vi "Number list to array.vi"(10 "Full names prefix":string, 11 "Number list":string) -> (2 "Full names":string[](array[string]), 3 "Number list array":i32[](array[numeric]))   [LabVIEW 2019]
panel:
  out "substring":string
  out "number":i32
  out "offset past number":i32
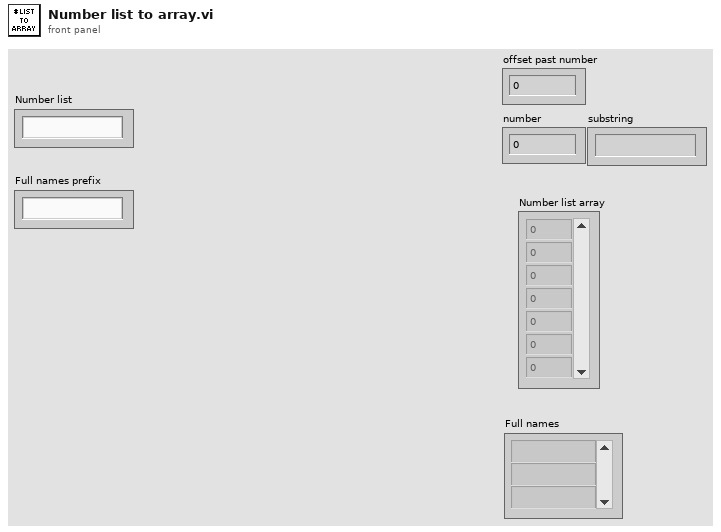
[diagram p1: front panel]
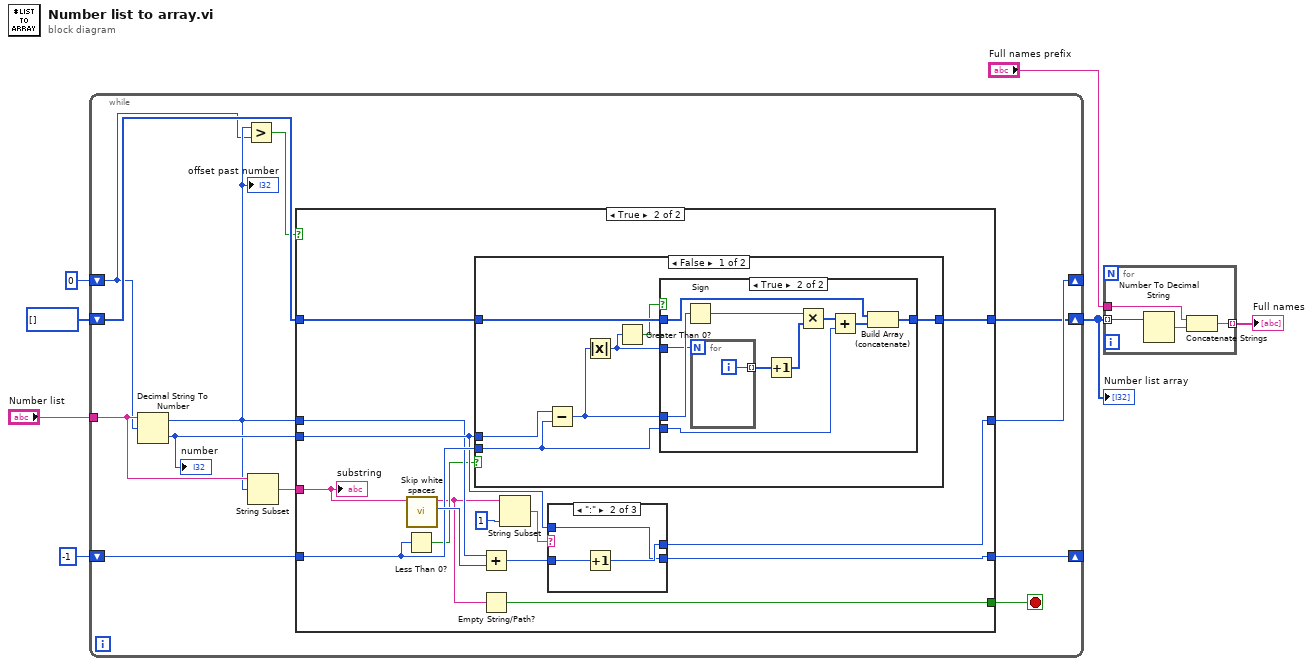
[diagram p0: block diagram]
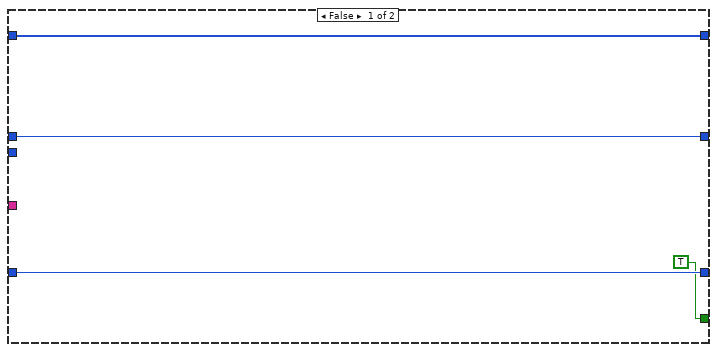
[diagram p2: hidden frame]
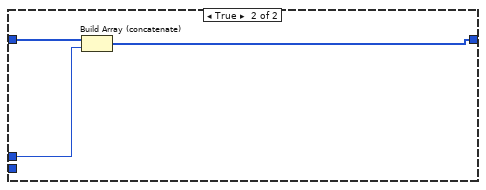
[diagram p4: hidden frame]
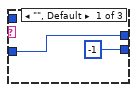
[diagram p5: hidden frame]
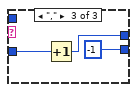
[diagram p6: hidden frame]
diagram:
  n1 = while {
    tunnel: "Number list" -> [w19]
    shift-right: [w11] -> w3
    shift-left: i32[] [] -> [w15]
    shift-right: [w17] -> _
    shift-left: 0 -> [w12]
    shift-right: [w9] -> _
    shift-left: -1 -> [w16]
    stop <- w8 stop-if-true
    n2 = Decimal String To Number(string=w19, offset=w12) -> (offset past number=w13:i32, number=w14:i32)  [unwired: 1 in]
    "offset past number" <- w13
    "number" <- w14
    n3 = Greater?(x=w13, y=w12) -> (0:w10:bool)
    n4 = String Subset(string=w19, offset (0)=w13) -> (substring=w18:string)  [unwired: 1 in]
    n5 = case shown="True" w10 {
      tunnel: w18 -> [_ w38]
      tunnel: [w21 w33] -> w17
      tunnel: w16 -> [w22 w32]
      tunnel: w15 -> [w23 w31]
      tunnel: w14 -> [_ w30]
      tunnel: w13 -> [w21 w29]
      tunnel: [w23 w28] -> w11
      tunnel: [w22 w26] -> w9
      tunnel: [TRUE w25] -> w8
      frame False {
      }
      frame True {
        n6 = Less Than 0?(x=w32) -> (x < 0?=w27:bool)
        n7 = call "Skip white spaces.vi"("String"=w38) -> ("1st non-white space"=w35:i32, "After white spaces"=w24:string)  [unwired: 9 in]
        n8 = case shown="False" w27 {
          tunnel: w31 -> [w42 w60]
          tunnel: [w41 w59] -> w28
          tunnel: w30 -> [w45 w58]
          tunnel: w32 -> [w43 _]
          frame False {
            n9 = Subtract(x=w45, y=w43) -> (x-y=w44:i32)
            n10 = Absolute Value(x=w44) -> (abs(x)=w40:i32)
            n11 = Greater Than 0?(x=w40) -> (x > 0?=w39:bool)
            n12 = case shown="True" w39 {
              tunnel: w44 -> [_ w55]
              tunnel: w40 -> [_ w54]
              tunnel: w43 -> [_ w51]
              tunnel: w42 -> [w46 w48]
              tunnel: [w46 w47] -> w41
              frame False {
              }
              frame True {
                n13 = Sign(1:w55) -> (0:w53:i32)
                n14 = for {
                  N: w54 -> [_]
                  tunnel: [w57] -> w56 mode=indexing
                  i -> [w57]
                }
                n15 = Increment(x=w56) -> (x+1=w52:i32[])
                n16 = Multiply(x=w53, y=w52) -> (x*y=w50:i32[])
                n17 = Add(x=w50, y=w51) -> (x+y=w49:i32[])
                n18 = Build Array (concatenate)(w48, w49) -> (w47:i32[])
              }
            }
          }
          frame True {
            n19 = Build Array (concatenate)(w60, w58) -> (w59:i32[])
          }
        }
        n20 = Add(x=w29, y=w35) -> (x+y=w34:i32)
        n21 = Empty String/Path?(string/path=w24) -> (empty?=w25:bool)
        n22 = String Subset(string=w24, length (rest)=1 ("length (rest)")) -> (substring=w36:string)  [unwired: 1 in]
        n23 = case shown="\":\"" w36 {
          tunnel: w30 -> [_ w63 _]
          tunnel: w34 -> [w62 w65 w68]
          tunnel: [w62 w64 w67] -> w33
          tunnel: [-1 w63 -1] -> w26
          frame "", Default {
          }
          frame ":" {
            n24 = Increment(x=w65) -> (x+1=w64:i32)
          }
          frame "," {
            n25 = Increment(x=w68) -> (x+1=w67:i32)
          }
        }
        "substring" <- w38
      }
    }
  }
  "Number list array" <- w3
  n26 = for {
    tunnel: w3 -> [w72] mode=indexing
    tunnel: [w70] -> w2 mode=indexing
    tunnel: "Full names prefix" -> [w69]
    n27 = Number To Decimal String(number=w72) -> (decimal integer string=w71:string)  [unwired: 1 in]
    n28 = Concatenate Strings(w69, w71) -> (w70:string)
  }
  "Full names" <- w2
